vi "CalabratedSteeringEncoder.vi"(1 "Steering Center":bool, 2 "Steer Encoder A":bool, 3 "Steer Encoder B":bool) -> (0 "f":i32)   [LabVIEW 2010]
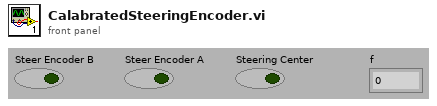
[diagram p1: front panel]
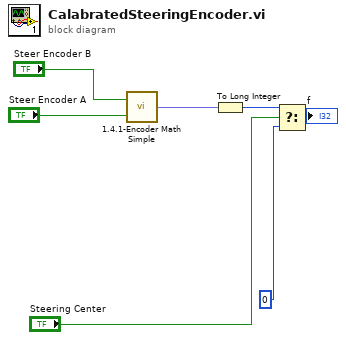
[diagram p0: block diagram]
diagram:
  n1 = call "1.4.1-Encoder Math Simple.vi"("B"="Steer Encoder A", "A"="Steer Encoder B") -> ("Numeric"=w3:fxp<+/-,2,2>)
  n2 = To Long Integer(number=w3) -> (32bit integer=w5:i32)
  n3 = Select(t=w5, s="Steering Center", f=0) -> (s? t:f=→"f":i32)
